vi "PictureLoop.vi"() -> ()   [LabVIEW 2017]
uses:
  TypeDefs/Position-Info-TD.ctl
  TypeDefs/Trav-Command-TD.ctl
  <vilib>/Utility/file.llb/Read Delimited Spreadsheet (I64).vi
  Settings/Traverse-Settings-Global.vi
panel:
  out "output cluster":T1
  out "Position Info OUT":T1
  in  "Trav Command":T2 items=["Set Reference", "Read Position", "Move"]
  in  "Position Info IN":T1
  out "Array":path[](array[path])
  out "all rows":i64[][](array[numeric])
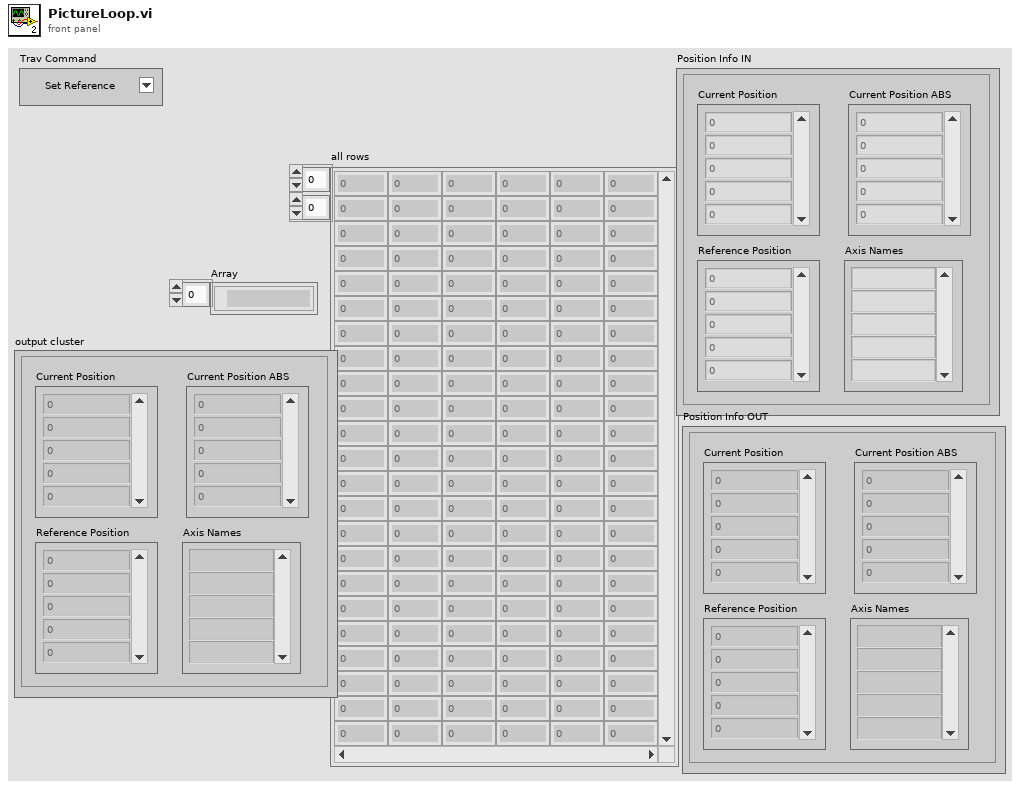
[diagram p1: front panel]
types:
  T1 = typedef "Position-Info-TD.ctl" = cluster{"Current Position ABS":dbl[], "Current Position":dbl[], "Reference Position":dbl[], "Axis Names":string[]}
  T2 = typedef "Trav-Command-TD.ctl" = u16
  T3 = typedef "Settings-Control.ctl" = cluster{"Acceleration":dbl[], "Deceleration":dbl[], "Max Velocity":dbl[], "Speed":dbl, "Pulse/Degree":dbl, "Degre Factor":dbl[], "mm/rotation":dbl[], "Traverse Name":string}
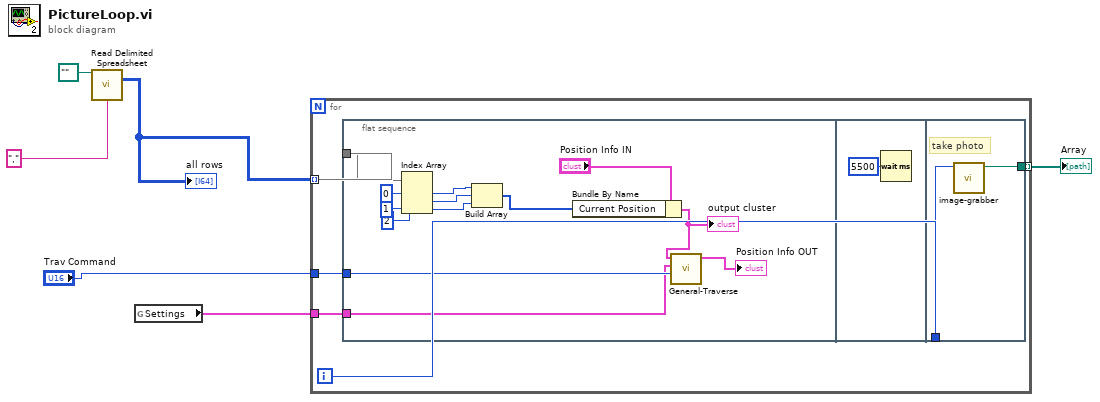
[diagram p0: block diagram]
diagram:
  n1 = call-poly <vilib>:"Read Delimited Spreadsheet.vi"("file path (dialog if empty)"=path "", "delimiter (\\t)"="," ("delimiter (\\t)")) -> ("all rows"=w3:i64[][])  [unwired: 8 in, 5 out]
  "all rows" <- w3
  n2 = global read "Traverse-Settings-Global.vi" "Settings"() -> (w1:T3)
  n3 = for {
    tunnel: w3 -> [w11] mode=indexing
    tunnel: [w10] -> w4 mode=indexing
    tunnel: "Trav Command" -> [w8]
    tunnel: w1 -> [w7]
    i -> [w9]
    n4 = flat-sequence {
      tunnel: w11 -> [w24]
      tunnel: w8 -> [w14]
      tunnel: w7 -> [w13]
      tunnel: w9 -> [w27]
      tunnel: [w26] -> w10
      frame #0 {
        n5 = Index Array(array=w24, index #1=0 ("index"), index #2=1 ("index"), index #3=2 ("index")) -> (element #1=w20:i64, element #2=w19:i64, element #3=w18:i64)
        n6 = Build Array(w20, w19, w18) -> (w16:i64[])
        n7 = Bundle By Name(cluster="Position Info IN", "Current Position"=w16) -> (w15:T1)
        "output cluster" <- w15
        n8 = call "General-Traverse.vi"("Trav Command"=w14, "Settings"=w13, "Position Info IN"=w15) -> ("Position Info OUT"=→"Position Info OUT":T1)  [unwired: 7 in, 1 out]
      }
      frame #1 {
        n9 = Wait (ms)(milliseconds to wait=u32 5500) -> ()  [unwired: 1 out]
      }
      frame #2 {
        # "take photo"
        n10 = call "image-grabber.vi"("Position number"=w27) -> ("Image path"=w26:path)  [unwired: 9 in, 1 out]
      }
    }
  }
  "Array" <- w4
